vi "GetLinkerDependencyFromFiles.vi"(9 "Overwrite LabVIEW Folder(If empty use this version of LabVIEW)":path, 11 "All Files in Dir":path[](array[path])) -> (3 "FileDependency":map{path, T1}(c390))   [LabVIEW 2020, in "DependencyChecker.lvlib"]
uses:
  DependencyChecker.lvlib
  FileDependencyType.ctl
  <vilib>/Utility/lvfile.llb/FT_FileTypes.ctl
  fa84a50a-7a91-41f1-93a7-6c8b41b91fd3.vi
  <vilib>/Utility/lvfile.llb/NI_FileType.lvlib
panel:
  in  "x":path
  out "Dependecy":T1
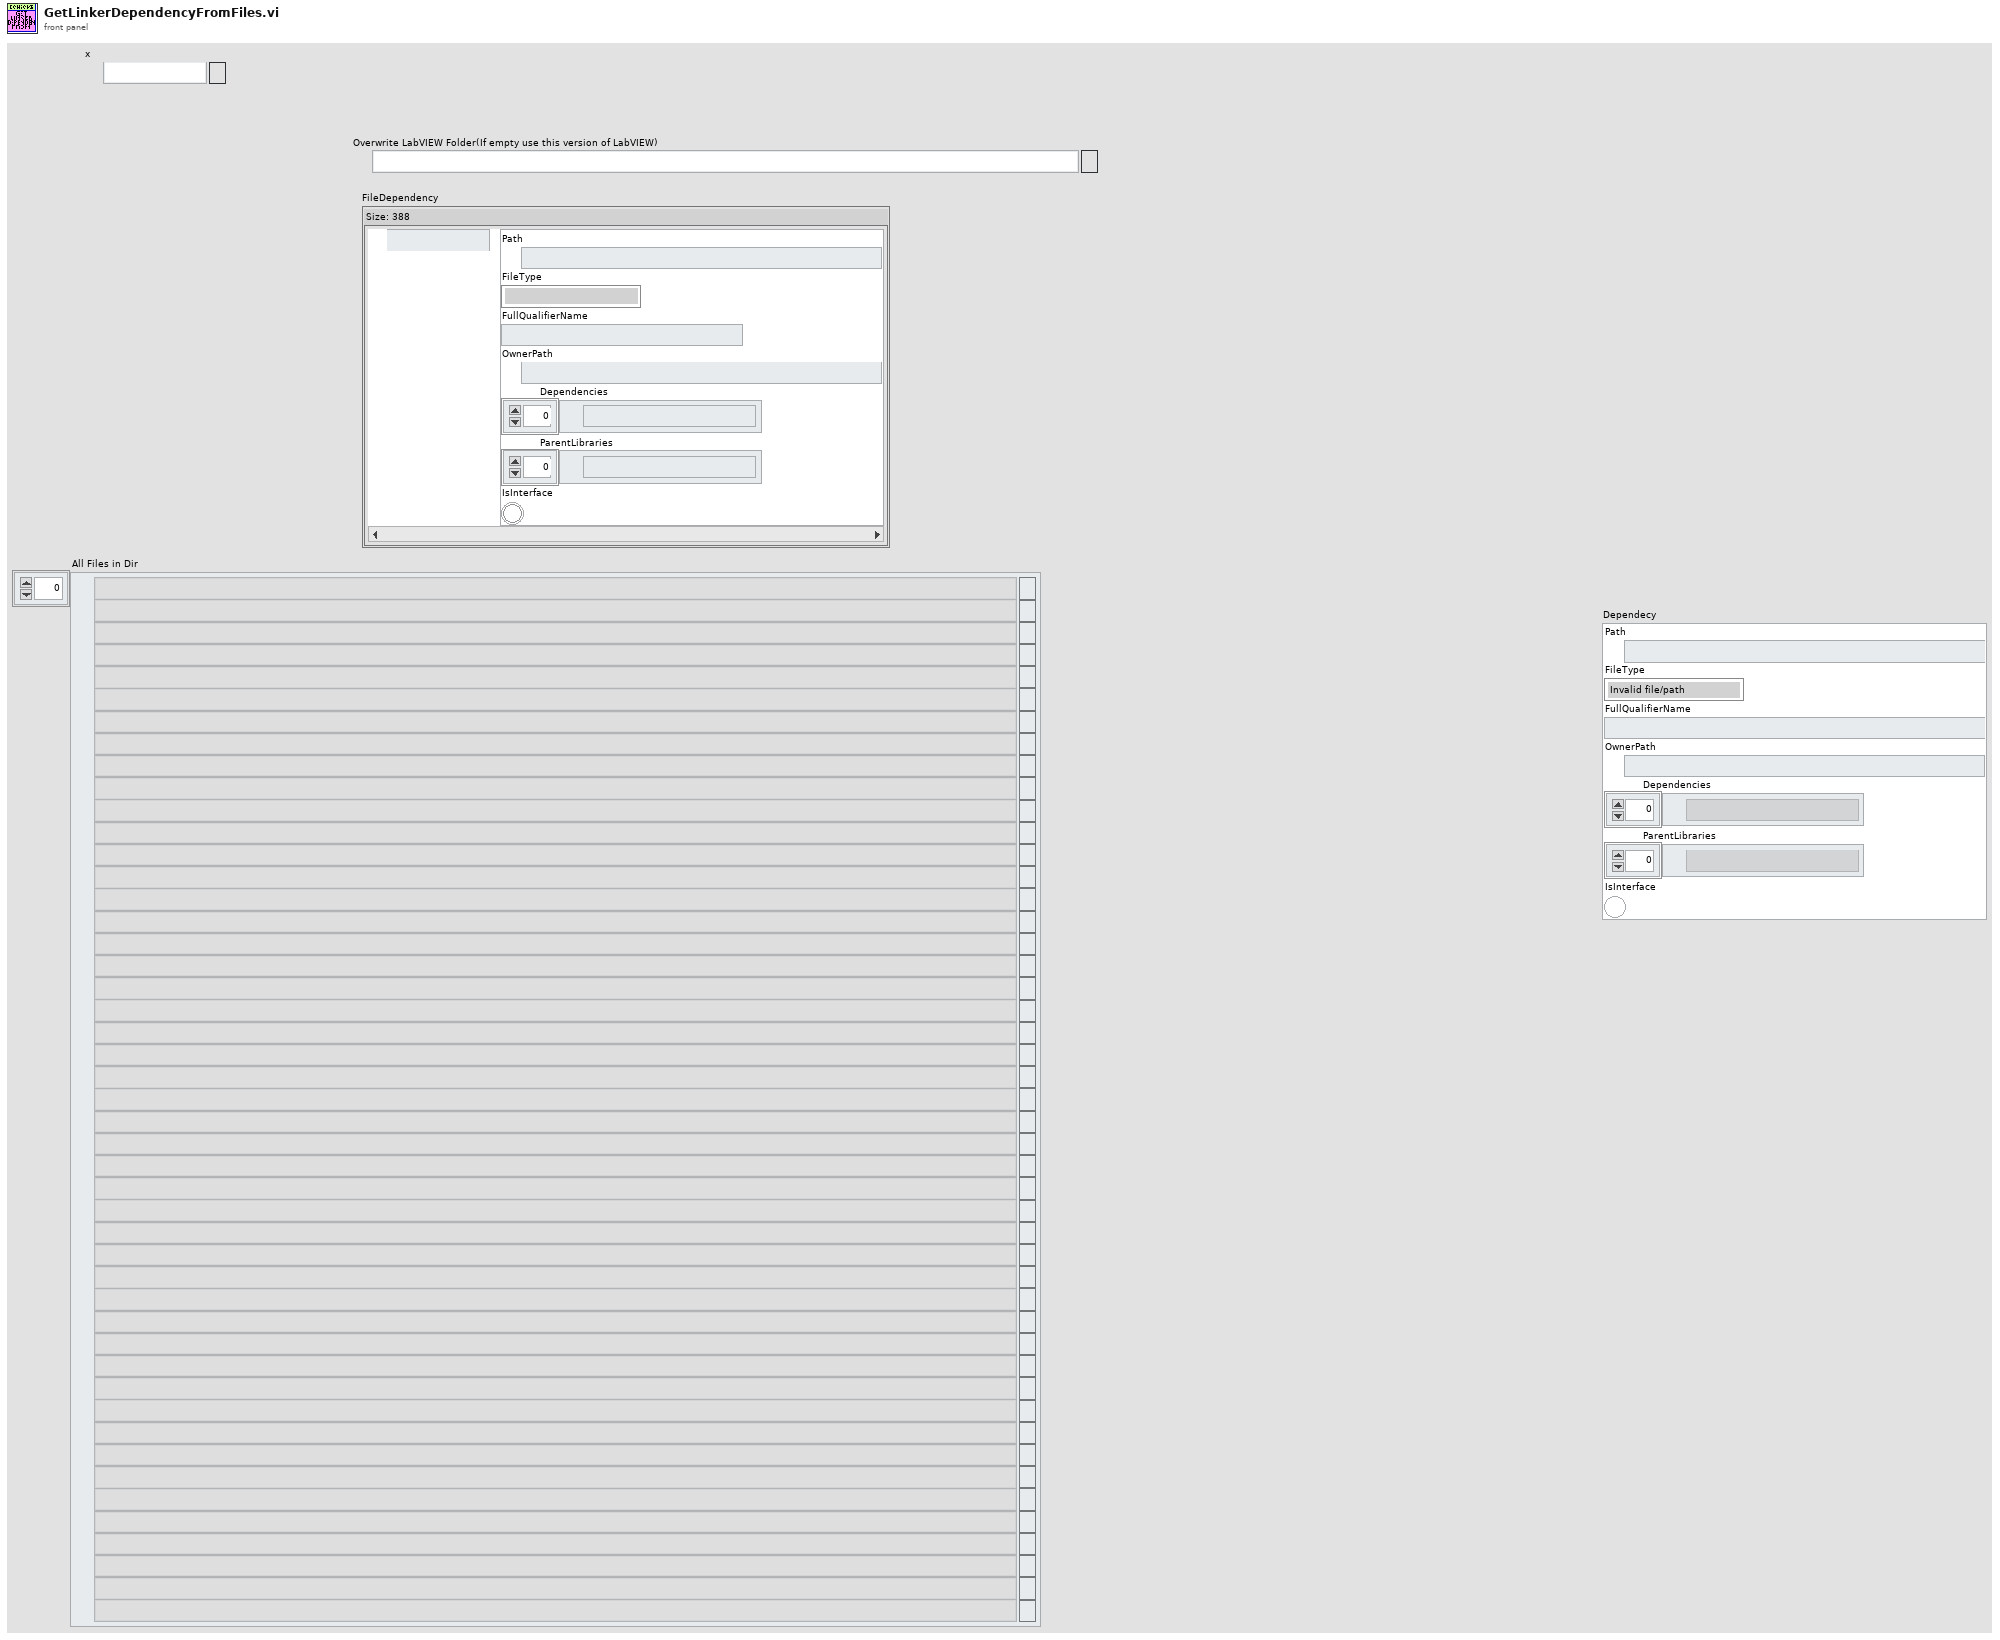
[diagram p1: front panel]
types:
  T1 = typedef "DependencyChecker.lvlib/FileDependencyType.ctl" = cluster{"Path":path, "FileType":T2, "FullQualifierName":string, "OwnerPath":path, "Dependencies":path[], "ParentLibraries":path[], "IsInterface":bool}
  T2 = typedef "NI_FileType.lvlib/FT_FileTypes.ctl" = enum32{"Invalid file/path", "Unknown type", "Instrument", "Control", "Polymorphic VI", "Project", "Library", "LVClass", "XControl", "XNode", "CIN", "Run-time menu", "Palette menu", "LLB", "Shortcut", "Directory", "Class Private Data Control", "Statechart", "MathScript .m file", "Ladder Diagram", "LVLibp"}
  T3 = typedef "NI_FileType.lvlib/LVFileType.ctl" = enum32{"Invalid file", "Unknown type", "Instrument", "Control", "Polymorphic VI", "Project", "Library", "LVClass", "XControl", "XNode", "Shared library", ".NET assembly", "ActiveX interface", "CIN", "Run-time menu", "Palette menu", "Help file", "LLB", "XNode Edit Dependency", "Class Private Data Control", "Statechart", "MathScript .m file", "Ladder Diagram", "LVLibp", "XNode Build Dependency"}
  T4 = cluster{"path":path, "delimited name":string, "type":T3, "iState":u32, "iStyle":u16, "wStyle":u16, "buttons":u16, "viflags":u32, "viflags2":u32, "links":u32[]}[]
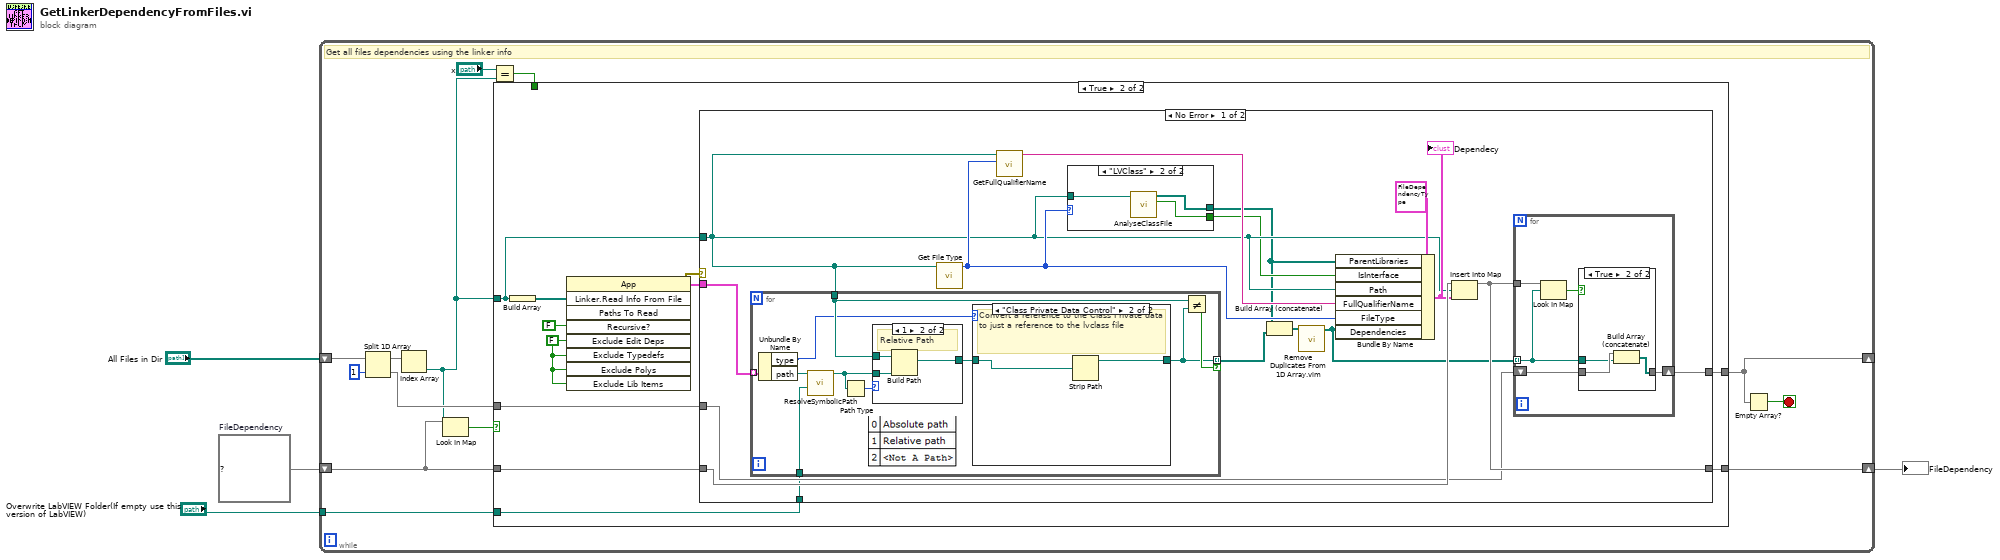
[diagram p0: block diagram]
diagram:
  w3 = map{path, T1} {}  # FileDependency
  n1 = while {
    shift-right: [w13] -> w4
    shift-left: w3 -> [w10]
    shift-right: [w11] -> _
    shift-left: "All Files in Dir" -> [w17]
    tunnel: "Overwrite LabVIEW Folder(If empty use this version of LabVIEW)" -> [w5]
    stop <- w12 stop-if-true
    # "Get all files dependencies using the linker info"
    n2 = Split 1D Array(array=w17, index=1) -> (first subarray=w15:path[], second subarray=w14:path[])
    n3 = Index Array(array=w15) -> (element=w8:path)  [unwired: 1 in]
    n4 = Look In Map(map=w10, key=w8) -> (key not found?=w9:bool)  [unwired: 1 in, 1 out]
    n5 = Equal?(x="x", y=w8) -> (x = y?=w6:bool)
    n6 = case shown="True" w9 {
      tunnel: w14 -> [w18 w30]
      tunnel: [w19 w29] -> w13
      tunnel: [w18 w28] -> w11
      tunnel: w10 -> [w19 w23]
      tunnel: w8 -> [_ w22]
      tunnel: w6 -> [_ _]
      tunnel: w5 -> [_ w20]
      frame False {
      }
      frame True {
        w21 = FALSE ("Exclude Edit Time Dependencies")
        n7 = Build Array(w22) -> (w27:path[])
        n8 = invoke class="App" method="Linker.Read Info From File"("Paths To Read"=w27, "Recursive?"=FALSE, "Exclude Edit Deps"=w21, "Exclude Typedefs"=w21, "Exclude Polys"=w21, "Exclude Lib Items"=w21) -> (error out=w24:errorcluster, "Linker.Read Info From File"=w25:T4)  [unwired: 3 in, 7 out]
        n9 = case shown="No Error" w24 {
          tunnel: w25 -> [w45 _]
          tunnel: w23 -> [w46 w76]
          tunnel: w30 -> [w42 w77]
          tunnel: [w41 w77] -> w28
          tunnel: w22 -> [w35 _]
          tunnel: [w43 w76] -> w29
          tunnel: w20 -> [w39 _]
          frame No Error {
            n10 = for {
              tunnel: w45 -> [w68] mode=indexing
              tunnel: [w59] -> w36 mode=indexing if=w65
              tunnel: w35 -> [w64]
              tunnel: w39 -> [w62]
              n11 = Unbundle By Name(w68) -> ("type"=w61:T3, "path"=w66:path)
              n12 = call "ResolveSymbolicPath.vi"("Overwrite LabVIEW Folder(If empty use this version of LabVIEW)"=w62, "path"=w66) -> ("File Path"=w63:path)  [unwired: 9 in]
              n13 = Path Type(1:w63) -> (0:w67:i16)
              n14 = case shown="1" w67 {
                tunnel: w63 -> [w72 w75]
                tunnel: [w72 w73] -> w60
                tunnel: w64 -> [_ w74]
                frame 0, Default {
                  # "Absolute Path"
                }
                frame 1 {
                  # "Relative Path"
                  n15 = Build Path(base path=w74, name or relative path=w75) -> (appended path=w73:path)
                }
              }
              n16 = case shown="\"Class Private Data Control\"" w61 {
                tunnel: w60 -> [w69 w71]
                tunnel: [w69 w70] -> w59
                frame Default {
                }
                frame "Class Private Data Control" {
                  # "Convert a reference to the Class Private data to just a reference to the lvclass file"
                  n17 = Strip Path(path=w71) -> (stripped path=w70:path)  [unwired: 1 out]
                }
              }
              n18 = Not Equal?(x=w64, y=w59) -> (x != y?=w65:bool)
            }
            n19 = call <vilib>:"Get File Type.vi"("path"=w35) -> ("file type"=w38:T2)  [unwired: 8 in, 2 out]
            n20 = call "GetFullQualifierName.vi"("file type"=w38, "File Path"=w35) -> ("FullQualifierName"=w40:string)  [unwired: 9 in]
            n21 = case shown="\"LVClass\"" w38 {
              tunnel: w35 -> [_ w49]
              tunnel: [_ w48] -> w33
              tunnel: [_ w47] -> w34
              frame "Invalid file/path", Default {
              }
              frame "LVClass" {
                n22 = call "AnalyseClassFile.vi"("File Path"=w49) -> ("IsInterface"=w47:bool, "ParentLibraries"=w48:path[])  [unwired: 9 in]
              }
            }
            n23 = Build Array (concatenate)(w33, w36) -> (w32:path[])
            n24 = call "Remove Duplicates From 1D Array.vim"("array"=w32) -> ("array with duplicates removed"=w31:path[])  [unwired: 10 in]
            n25 = Bundle By Name(cluster=T1 {"Path"=path "", "FileType"=enum."Instrument", "FullQualifierName"="Decorator1_Main.vi", "OwnerPath"=path "", "Dependencies"=[], "ParentLibraries"=[], "IsInterface"=FALSE} ("value"), "ParentLibraries"=w33, "IsInterface"=w34, "Path"=w35, "FullQualifierName"=w40, "FileType"=w38, "Dependencies"=w31) -> (w44:T1)
            "Dependecy" <- w44
            n26 = Insert Into Map(map in=w46, key=w35, value=w44) -> (map out=w43:map{path, T1})  [unwired: 2 out]
            n27 = for {
              tunnel: w43 -> [w54]
              tunnel: w31 -> [w50] mode=indexing
              shift-right: [w51] -> w41
              shift-left: w42 -> [w52]
              n28 = Look In Map(map=w54, key=w50) -> (key not found?=w53:bool)  [unwired: 1 in, 1 out]
              n29 = case shown="True" w53 {
                tunnel: w52 -> [w55 w58]
                tunnel: [w55 w57] -> w51
                tunnel: w50 -> [_ w56]
                frame False {
                }
                frame True {
                  n30 = Build Array (concatenate)(w58, w56) -> (w57:path[])
                }
              }
            }
          }
          frame Error {
          }
        }
      }
    }
    n31 = Empty Array?(array=w11) -> (empty?=w12:bool)
  }
  "FileDependency" <- w4
